vi "ArrayAverage.vi"(11 "array":dbl[](array[numeric])) -> (3 "Average":dbl)   [LabVIEW 2013]
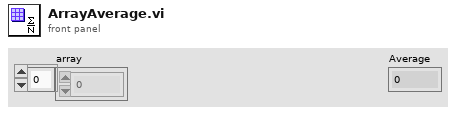
[diagram p1: front panel]
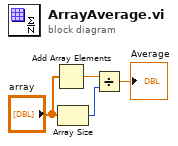
[diagram p0: block diagram]
diagram:
  n1 = Add Array Elements(numeric array="array") -> (sum=w1:dbl)
  n2 = Array Size(array="array") -> (size(s)=w4:i32)
  n3 = Divide(x=w1, y=w4) -> (x/y=→"Average":dbl)
